vi "DriveReadEncoder.vi"(11 "ModualNamePrefix":string) -> ()   [LabVIEW 2020]
uses:
  <vilib>/Rock Robotics/Network Tables/NT Write Number.vi
  <vilib>/Rock Robotics/WPI/ThirdParty/Phoenix-LabVIEW/CANCoder/Get/CTRE_Phoenix_CANcoder_GetSensorData.vi
panel:
  out "error out":errorcluster
  in  "error in":errorcluster
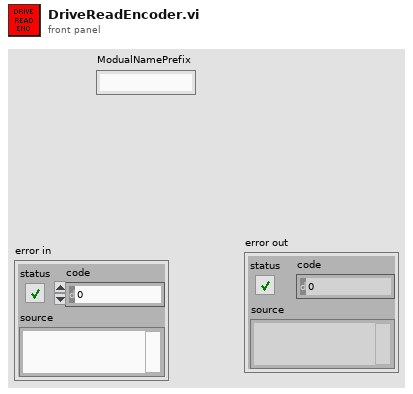
[diagram p1: front panel]
types:
  T1 = typedef "CTRE_Phoenix_CANcoder_DeviceRef.ctl" = cluster{"DeviceStatus":errorcluster, "Device Number":u8, "Handle":u64, "UsageFrame":u32, "Library Path":path}
  T2 = typedef "WPI_MotorControlDeviceRef.ctl" = cluster{"DeviceStatus":errorcluster, "Type":T3, "PWM":cluster{"PWM Channel":T4, "DeadBand":T5}, "CAN":cluster{"Device Number":u8, "SetOutput VI Ref":variant, "GetOutput VI Ref":variant, "Enable VI Ref":variant, "Disable VI Ref":variant, "Data":variant}, "Invert":bool, "DIO PWM":cluster{"PWM \"Enable\" Channel":T4, "DIOChannel":T6, "PWM Rate":dbl}}
  T3 = typedef "WPI_MotorControlType.ctl" = enum16{"PWM", "CAN", "DIO PWM"}
  T4 = typedef "FPGA_DIOPWMChannel.ctl" = enum8{"PWM 0", "PWM 1", "PWM 2", "PWM 3", "PWM 4", "PWM 5", "PWM 6", "PWM 7", "PWM 8", "PWM 9", "PWM MXP 0", "PWM MXP 1", "PWM MXP 2", "PWM MXP 3", "PWM MXP 4", "PWM MXP 5", "PWM MXP 6", "PWM MXP 7", "PWM MXP 8", "PWM MXP 9", "Invalid"}
  T5 = typedef "WPI_PWMDeadband.ctl" = cluster{"Name":string, "maxPositivePwm":i32, "minPositivePwm":i32, "centerPwm":i32, "maxNegativePwm":i32, "minNegativePwm":i32, "angularRange":u16}
  T6 = typedef "FPGA_DIOChannel.ctl" = enum8{"DIO 0", "DIO 1", "DIO 2", "DIO 3", "DIO 4", "DIO 5", "DIO 6", "DIO 7", "DIO 8", "DIO 9", "DIO MXP 0", "DIO MXP 1", "DIO MXP 2", "DIO MXP 3", "DIO MXP 4", "DIO MXP 5", "DIO MXP 6", "DIO MXP 7", "DIO MXP 8", "DIO MXP 9", "DIO MXP 10", "DIO MXP 11", "DIO MXP 12", "DIO MXP 13", "DIO MXP 14", "DIO MXP 15", "SPI Port CS1", "SPI Port CS2", "SPI Port CS3", "SPI Port MISO", "SPI Port MOSI", "Invalid"}
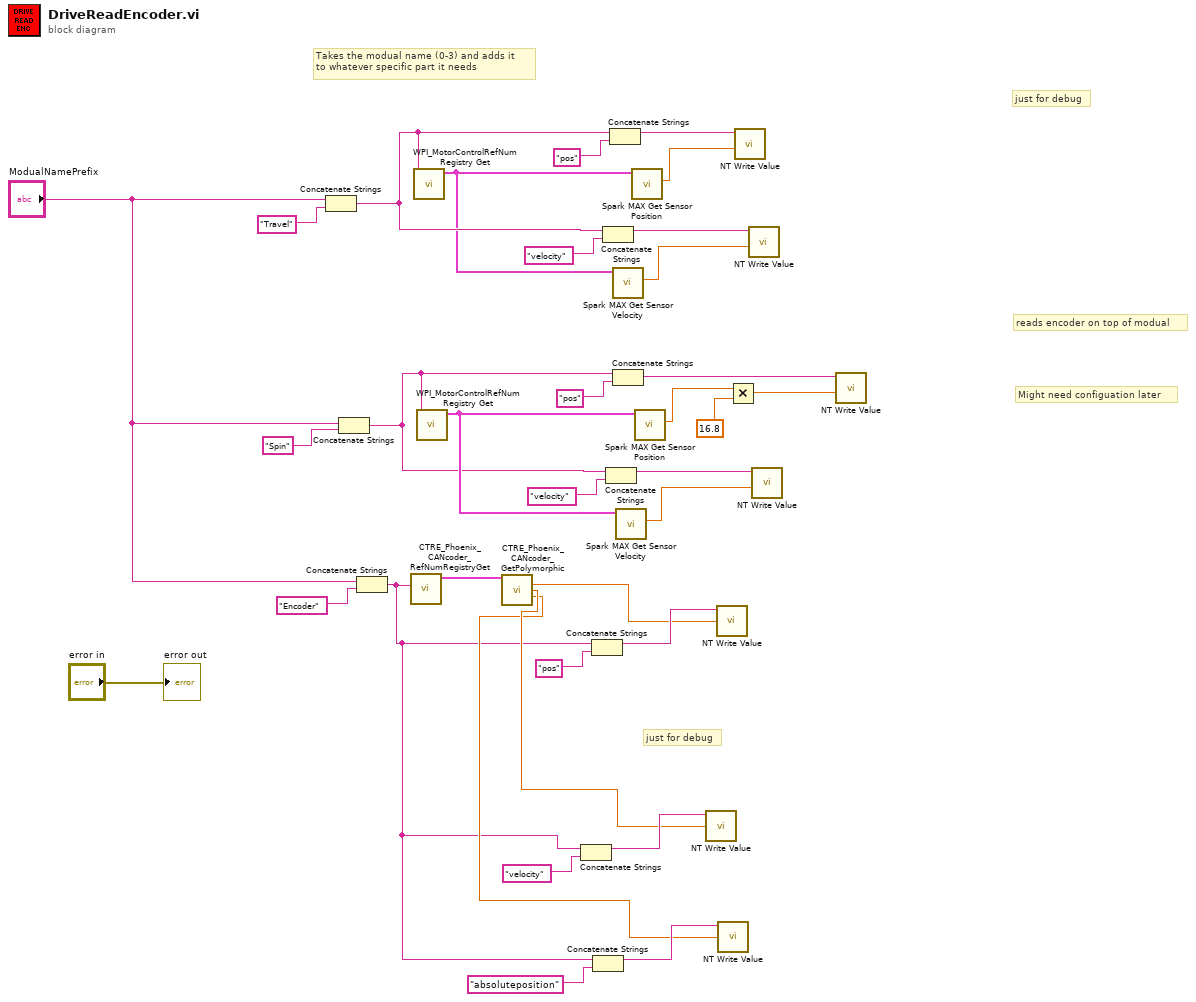
[diagram p0: block diagram]
diagram:
  # "just for debug"
  # "just for debug"
  # "reads encoder on top of modual"
  # "Might need configuation later"
  # "Takes the modual name (0-3) and adds it \nto whatever specific part it needs"
  n1 = Concatenate Strings("ModualNamePrefix", "Travel" ("refnum name")) -> (w14:string)
  n2 = Concatenate Strings("ModualNamePrefix", "Spin" ("refnum name")) -> (w4:string)
  n3 = Concatenate Strings("ModualNamePrefix", "Encoder" ("refnum name")) -> (w19:string)
  n4 = call <vilib>:"CTRE_Phoenix_CANcoder_RefNumRegistryGet.vi"("refnum name"=w19) -> ("CTRE_CANcoder_DeviceRef"=w29:T1)  [unwired: 9 in, 1 out]
  n5 = call <vilib>:"WPI_MotorControlRefNum Registry Get.vi"("refnum name"=w14) -> ("MotorControlDevRef"=w13:T2)  [unwired: 9 in, 1 out]
  n6 = call <vilib>:"WPI_MotorControlRefNum Registry Get.vi"("refnum name"=w4) -> ("MotorControlDevRef"=w6:T2)  [unwired: 9 in, 1 out]
  n7 = call-poly <vilib>:"CTRE_Phoenix_CANcoder_GetPolymorphic.vi"("CTRE_CANcoder_DeviceRef"=w29) -> ("Position"=w26:dbl, "Velocity"=w21:dbl, "Absolute Position"=w20:dbl)  [unwired: 10 in, 2 out]
  n8 = Concatenate Strings(w19, "velocity" ("refnum name")) -> (w24:string)
  n9 = Concatenate Strings(w19, "pos" ("refnum name")) -> (w27:string)
  n10 = Concatenate Strings(w19, "absoluteposition" ("refnum name")) -> (w22:string)
  n11 = Concatenate Strings(w14, "velocity" ("refnum name")) -> (w15:string)
  n12 = Concatenate Strings(w4, "velocity" ("refnum name")) -> (w7:string)
  n13 = Concatenate Strings(w14, "pos" ("refnum name")) -> (w17:string)
  n14 = call <vilib>:"Spark MAX Get Sensor Velocity.vi"("MotorControlDevRef in"=w13) -> ("Sensor Velocity"=w12:dbl)  [unwired: 7 in, 3 out]
  n15 = Concatenate Strings(w4, "pos" ("refnum name")) -> (w9:string)
  n16 = call <vilib>:"Spark MAX Get Sensor Velocity.vi"("MotorControlDevRef in"=w6) -> ("Sensor Velocity"=w5:dbl)  [unwired: 7 in, 3 out]
  n17 = call <vilib>:"Spark MAX Get Sensor Position.vi"("MotorControlDevRef in"=w13) -> ("Sensor Position"=w11:dbl)  [unwired: 7 in, 3 out]
  n18 = call <vilib>:"Spark MAX Get Sensor Position.vi"("MotorControlDevRef in"=w6) -> ("Sensor Position"=w3:dbl)  [unwired: 7 in, 3 out]
  n19 = call-poly <vilib>:"NT Write Value.vi"("value"=w21, "name"=w24) -> ()  [unwired: 9 in, 1 out]
  n20 = call-poly <vilib>:"NT Write Value.vi"("value"=w26, "name"=w27) -> ()  [unwired: 9 in, 1 out]
  n21 = call-poly <vilib>:"NT Write Value.vi"("value"=w20, "name"=w22) -> ()  [unwired: 9 in, 1 out]
  n22 = Multiply(x=w3, y=16.8) -> (x*y=w1:dbl)
  n23 = call-poly <vilib>:"NT Write Value.vi"("value"=w11, "name"=w17) -> ()  [unwired: 9 in, 1 out]
  n24 = call-poly <vilib>:"NT Write Value.vi"("value"=w12, "name"=w15) -> ()  [unwired: 9 in, 1 out]
  n25 = call-poly <vilib>:"NT Write Value.vi"("value"=w5, "name"=w7) -> ()  [unwired: 9 in, 1 out]
  n26 = call-poly <vilib>:"NT Write Value.vi"("value"=w1, "name"=w9) -> ()  [unwired: 9 in, 1 out]
  "error out" <- "error in"
